vi "Ordenar Lista de controladores.vi"(0 "subarray":string[][](array[string]), 5 "error in (no error)":errorcluster) -> (10 "3D Ordered array":string[][][](array[string]), 11 "Sorted 2D table array":string[][](array[string]), 19 "error out":errorcluster)   [LabVIEW 2019]
uses:
  9384e772-f1e9-4660-a55d-f0fb9543d4e1.vi
  <vilib>/Array/Sort 2D Array - Pop Stack.vi
  <vilib>/Array/Sort 2D Array - Push Stack.vi
  Variable global de carga.vi
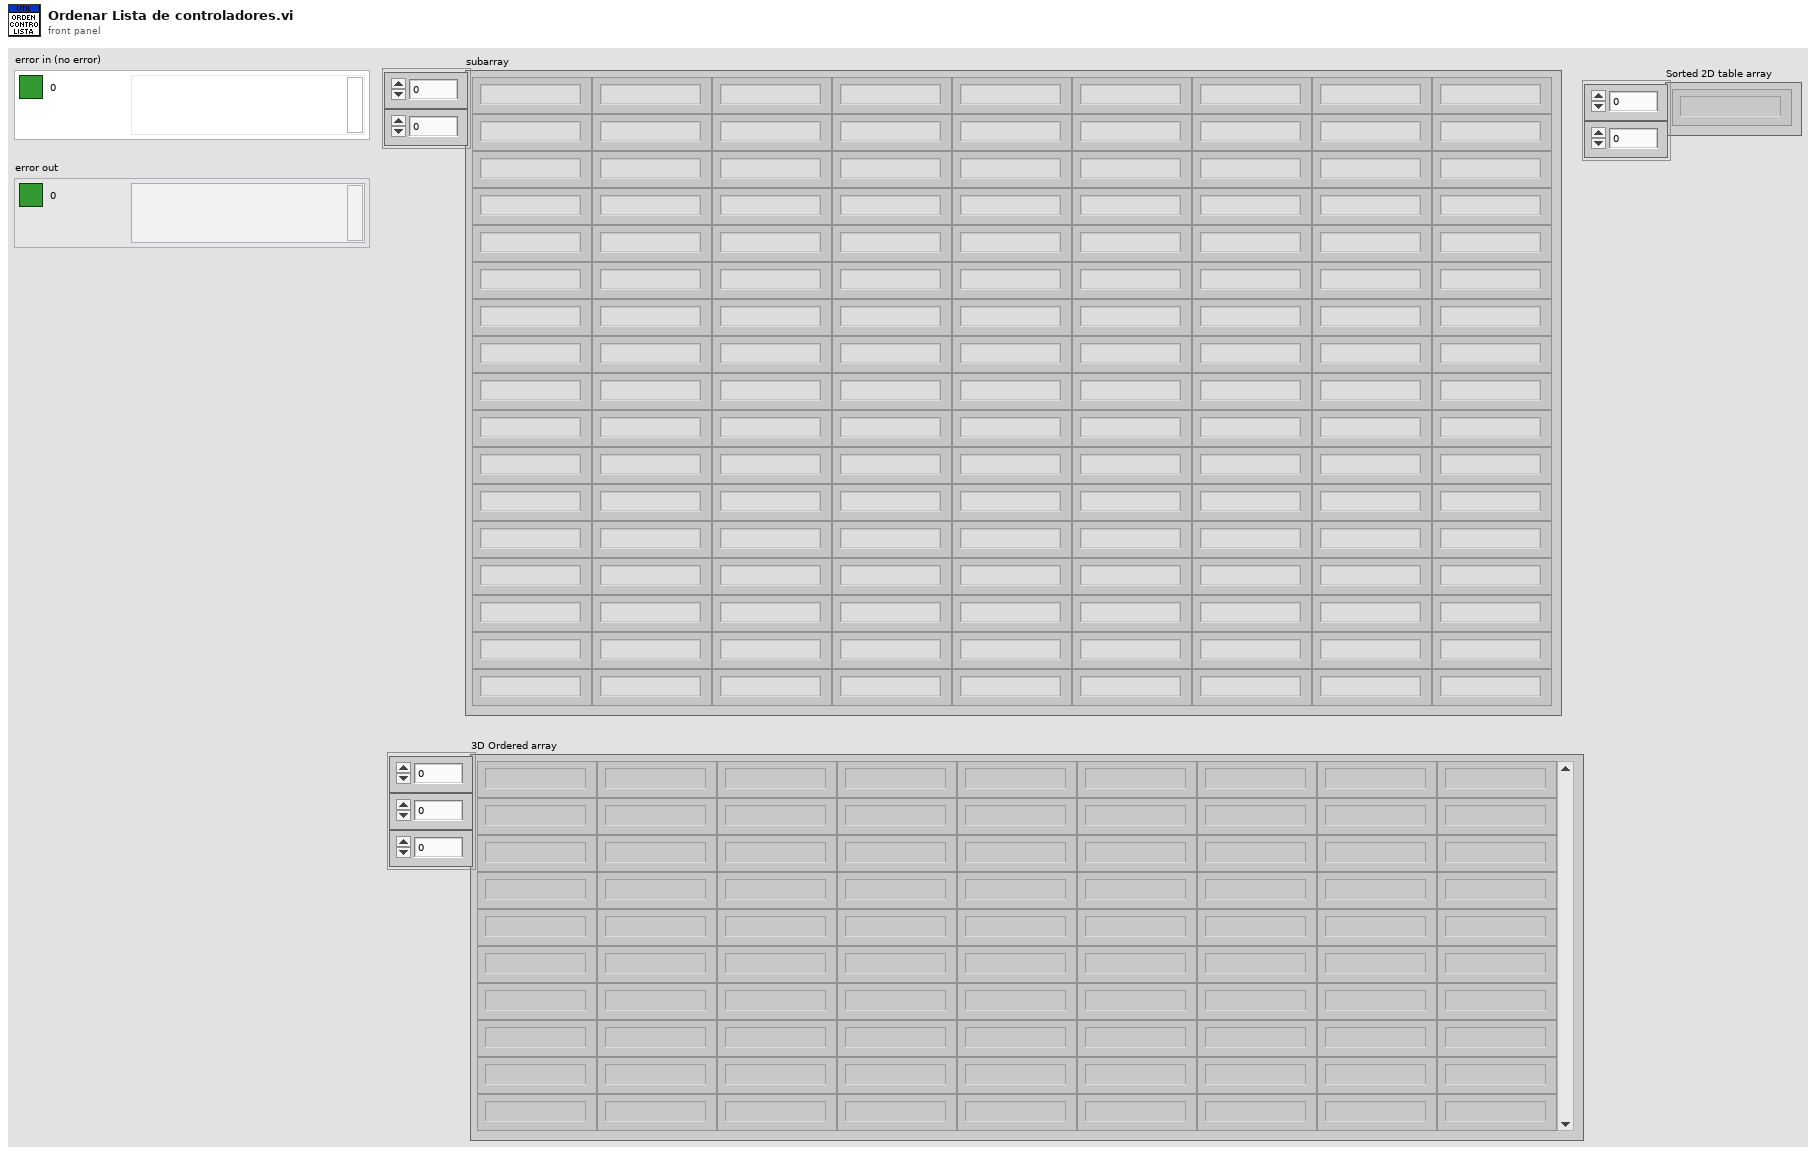
[diagram p1: front panel]
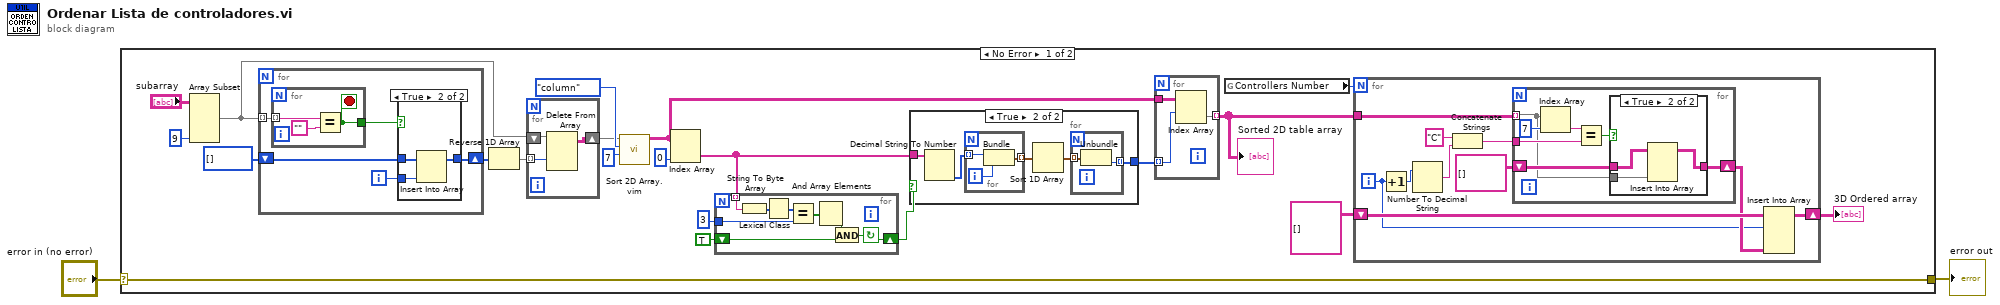
[diagram p0: block diagram]
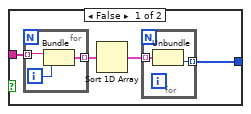
[diagram p3: hidden frame]
diagram:
  n1 = case shown="No Error" "error in (no error)" {
    selector: "error in (no error)" -> [w23 w90]
    tunnel: [w23 w90] -> w1
    frame No Error {
      n2 = Array Subset(array="subarray", length (col)=9 ("length")) -> (w15:string[][])  [unwired: 3 in]
      n3 = for {
        tunnel: w15 -> [w82] mode=indexing
        shift-right: [w78] -> w18
        shift-left: i32[] [] -> [w79]
        i -> [w81]
        n4 = for {
          tunnel: w82 -> [w89] mode=indexing
          tunnel: [w87] -> w80
          stop <- w87 stop-if-true
          n5 = Equal?(x=w89, y="") -> (x = y?=w87:bool)
        }
        n6 = case shown="True" w80 {
          tunnel: w81 -> [_ w86]
          tunnel: w79 -> [w83 w85]
          tunnel: [w83 w84] -> w78
          frame False {
          }
          frame True {
            n7 = Insert Into Array(array=w85, new element=w86) -> (w84:i32[])  [unwired: 1 in]
          }
        }
      }
      n8 = Reverse 1D Array(array=w18) -> (reversed array=w17:i32[])
      n9 = for {
        tunnel: w17 -> [w77] mode=indexing
        shift-right: [w75] -> w20
        shift-left: w15 -> [w76]
        n10 = Delete From Array(array=w76, index (row)=w77) -> (array with subset deleted=w75:string[][])  [unwired: 2 in, 1 out]
      }
      n11 = call "Sort 2D Array.vim"("index"=7, "dimension to index (column)"=enum16{"column", "row"}."column", "2D array"=w20) -> ("sorted 2D array"=w8:string[][])  [unwired: 7 in, 1 out]
      n12 = Index Array(array=w8, index (col)=0) -> (element=w12:string[])  [unwired: 1 in]
      n13 = for {
        tunnel: w12 -> [w74] mode=indexing
        tunnel: i16 3 ("y") -> [w73]
        shift-right: [w67] -> w9
        shift-left: TRUE -> [w68]
        stop <- w67 continue-if-true
        n14 = String To Byte Array(string=w74) -> (unsigned byte array=w71:u8[])
        n15 = Lexical Class(1:w71) -> (0:w72:i16[])
        n16 = Equal?(x=w72, y=w73) -> (x = y?=w70:bool[])
        n17 = And Array Elements(Boolean array=w70) -> (logical AND=w69:bool)
        n18 = And(x=w69, y=w68) -> (x .and. y?=w67:bool)
      }
      n19 = case shown="True" w9 {
        tunnel: w12 -> [w48 w58]
        tunnel: [w45 w54] -> w13
        frame False {
          n20 = for {
            tunnel: w48 -> [w52] mode=indexing
            tunnel: [w51] -> w47 mode=indexing
            i -> [w53]
            n21 = Bundle("String"=w52, w53) -> (w51:cluster{"String":string, i32})  [unwired: 1 in]
          }
          n22 = Sort 1D Array(array=w47) -> (sorted array=w46:cluster{"String":string, i32}[])
          n23 = for {
            tunnel: w46 -> [w50] mode=indexing
            tunnel: [w49] -> w45 mode=indexing
            n24 = Unbundle(w50) -> (w49:i32)  [unwired: 1 out]
          }
        }
        frame True {
          n25 = Decimal String To Number(string=w58) -> (number=w57:i32[])  [unwired: 2 in, 1 out]
          n26 = for {
            tunnel: w57 -> [w62] mode=indexing
            tunnel: [w61] -> w56 mode=indexing
            i -> [w63]
            n27 = Bundle("String"=w62, w63) -> (w61:cluster{"String":i32, i32})  [unwired: 1 in]
          }
          n28 = Sort 1D Array(array=w56) -> (sorted array=w55:cluster{"String":i32, i32}[])
          n29 = for {
            tunnel: w55 -> [w60] mode=indexing
            tunnel: [w59] -> w54 mode=indexing
            n30 = Unbundle(w60) -> (w59:i32)  [unwired: 1 out]
          }
        }
      }
      n31 = for {
        tunnel: w8 -> [w66]
        tunnel: w13 -> [w65] mode=indexing
        tunnel: [w64] -> w6 mode=indexing
        n32 = Index Array(array=w66, index (row)=w65) -> (element=w64:string[])  [unwired: 1 in]
      }
      "Sorted 2D table array" <- w6
      n33 = global read "Variable global de carga.vi" "Controllers Number"() -> (w5:u16)
      n34 = for {
        N: w5 -> [_]
        tunnel: w6 -> [w33]
        shift-right: [w26] -> w3
        shift-left: string[][][] [] -> [w27]
        i -> [w24]
        n35 = Increment(x=w24) -> (x+1=w31:i32)
        n36 = Number To Decimal String(number=w31) -> (decimal integer string=w30:string)  [unwired: 1 in]
        n37 = Concatenate Strings("C", w30) -> (w29:string)
        n38 = for {
          tunnel: w33 -> [w35] mode=indexing
          tunnel: w29 -> [w38]
          shift-right: [w34] -> w25
          shift-left: string[][] [] -> [w37]
          n39 = Index Array(array=w35, index=7) -> (element=w39:string)
          n40 = Equal?(x=w39, y=w38) -> (x = y?=w36:bool)
          n41 = case shown="True" w36 {
            tunnel: w37 -> [w41 w44]
            tunnel: w35 -> [_ w42]
            tunnel: [w41 w43] -> w34
            frame False {
            }
            frame True {
              n42 = Insert Into Array(array=w44, new element=w42) -> (w43:string[][])  [unwired: 2 in]
            }
          }
        }
        n43 = Insert Into Array(array=w27, index (dim 0)=w24, new element=w25) -> (w26:string[][][])  [unwired: 2 in]
      }
      "3D Ordered array" <- w3
    }
    frame Error {
    }
  }
  "error out" <- w1
